vi "Impulse sign and direction 2.vi"(3 "Threshold of either torsion or pitch velocity to determine RALP/LARP":dbl=30.0 format="%.2f", 5 "Peak X Y Z L R Values":dbl[](array[numeric]) format="%.2f") -> (2 "Impulse":T1)   [LabVIEW 2016, in "impulse functions.lvlib"]
uses:
  impulse functions.lvlib
panel:
  # "If the rotational component is more than half the vertical component in magnitude then this is a RALP/LARP stimulus"
  # "Copyright Americo A. Migliaccio (c) 2002 All Rights Reserved by Author"
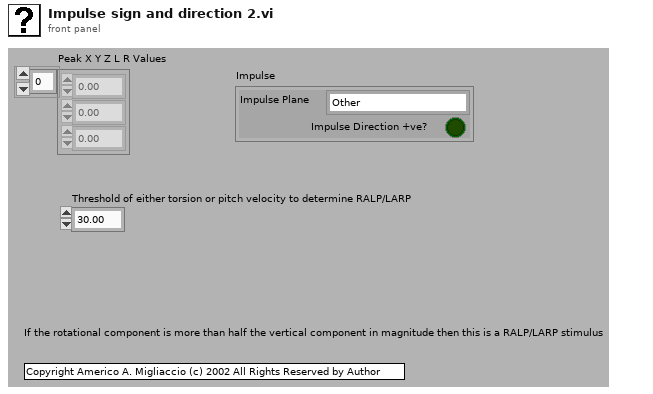
[diagram p1: front panel]
types:
  T1 = cluster{"Impulse Plane":enum16{"Other", "Yaw", "Pitch", "Roll", "LARP", "RALP"}, "Impulse Direction +ve?":bool}
  T2 = enum16{"Other", "Yaw", "Pitch", "Roll", "LARP", "RALP"}
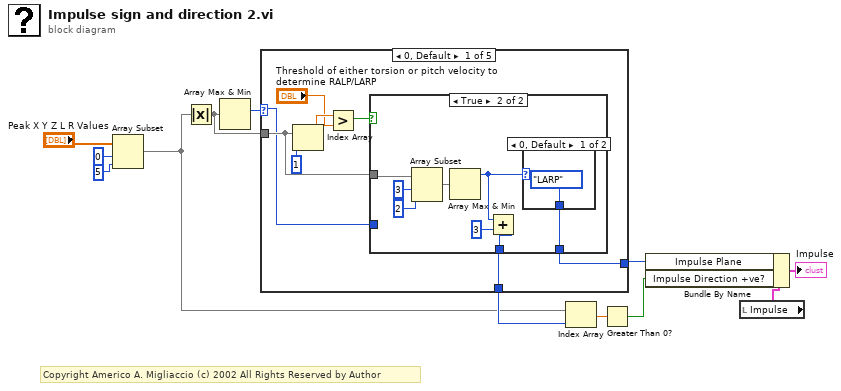
[diagram p0: block diagram]
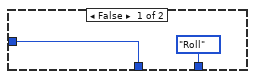
[diagram p2: hidden frame]
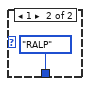
[diagram p3: hidden frame]
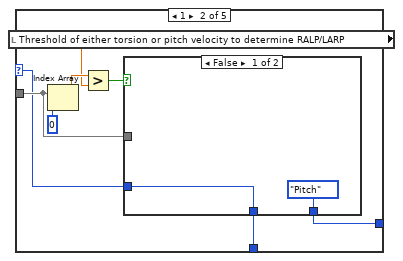
[diagram p4: hidden frame]
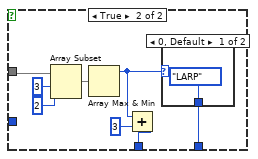
[diagram p5: hidden frame]
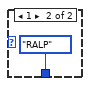
[diagram p6: hidden frame]
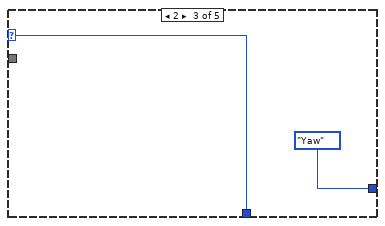
[diagram p7: hidden frame]
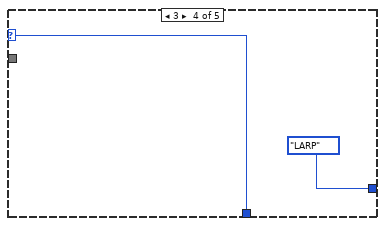
[diagram p8: hidden frame]
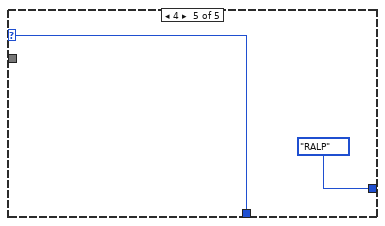
[diagram p9: hidden frame]
diagram:
  # "Copyright Americo A. Migliaccio (c) 2002 All Rights Reserved by Author"
  n1 = Array Subset(array="Peak X Y Z L R Values", index=0 ("Array Index"), length=5 ("Array Length")) -> (w2:dbl[])
  n2 = Absolute Value(x=w2) -> (abs(x)=w6:dbl[])
  n3 = Array Max & Min(array=w6) -> (max index (indices)=w1:i32)  [unwired: 3 out]
  n4 = case shown="0, Default" w1 {
    selector: w1 -> [w15 w34 w53 w55 w57]
    tunnel: [w13 w38 T2."Yaw" ("Impulse Plane") T2."LARP" ("Impulse Plane") T2."RALP" ("Impulse Plane")] -> w7
    tunnel: w6 -> [w16 w37 _ _ _]
    tunnel: [w14 w33 w53 w55 w57] -> w4
    frame 0, Default {
      n5 = Index Array(array=w16, index=1 ("Index")) -> (element=w19:dbl)
      n6 = Greater?(x=w19, y="Threshold of either torsion or pitch velocity to determine RALP/LARP") -> (0:w17:bool)
      n7 = case shown="True" w17 {
        tunnel: [T2."Roll" ("Impulse Plane") w27] -> w13
        tunnel: w16 -> [_ w30]
        tunnel: [w21 w23] -> w14
        tunnel: w15 -> [w21 _]
        frame False {
        }
        frame True {
          n8 = Array Subset(array=w30, index=3 ("Array Index"), length=2 ("Array Length")) -> (w26:dbl[])
          n9 = Array Max & Min(array=w26) -> (max index (indices)=w25:i32)  [unwired: 3 out]
          n10 = Add(x=w25, y=3) -> (x+y=w23:i32)
          n11 = case shown="0, Default" w25 {
            tunnel: [T2."LARP" ("Impulse Plane") T2."RALP" ("Impulse Plane")] -> w27
            frame 0, Default {
            }
            frame 1 {
            }
          }
        }
      }
    }
    frame 1 {
      n12 = local read "Threshold of either torsion or pitch velocity to determine RALP/LARP"() -> (w35:dbl)
      n13 = Index Array(array=w37, index=0 ("Index")) -> (element=w36:dbl)
      n14 = Greater?(x=w36, y=w35) -> (0:w39:bool)
      n15 = case shown="False" w39 {
        tunnel: [T2."Pitch" ("Impulse Plane") w47] -> w38
        tunnel: w37 -> [_ w50]
        tunnel: [w41 w43] -> w33
        tunnel: w34 -> [w41 _]
        frame False {
        }
        frame True {
          n16 = Array Subset(array=w50, index=3 ("Array Index"), length=2 ("Array Length")) -> (w46:dbl[])
          n17 = Array Max & Min(array=w46) -> (max index (indices)=w45:i32)  [unwired: 3 out]
          n18 = Add(x=w45, y=3) -> (x+y=w43:i32)
          n19 = case shown="0, Default" w45 {
            tunnel: [T2."LARP" ("Impulse Plane") T2."RALP" ("Impulse Plane")] -> w47
            frame 0, Default {
            }
            frame 1 {
            }
          }
        }
      }
    }
    frame 2 {
    }
    frame 3 {
    }
    frame 4 {
    }
  }
  n20 = Index Array(array=w2, index=w4) -> (element=w5:dbl)
  n21 = Greater Than 0?(x=w5) -> (x > 0?=w3:bool)
  n22 = local read "Impulse"() -> (w12:T1)
  n23 = Bundle By Name(cluster=w12, "Impulse Plane"=w7, "Impulse Direction +ve?"=w3) -> (→"Impulse":T1)
